vi "Check Condition.vi"(1 "Distance":dbl, 2 "Condition":dbl, 3 "Reset":bool) -> (0 "Done":bool)   [LabVIEW 2015]
uses:
  Robot Global Data.vi
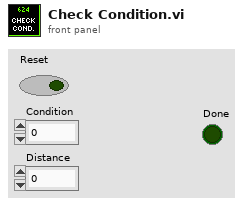
[diagram p1: front panel]
types:
  T1 = typedef "Encoder Values Super Cluster.ctl" = cluster{"Left Encoder":T2, "Right Encoder":T2}
  T2 = typedef "Encoder Values.ctl" = cluster{"Distance":dbl, "Speed":dbl, "Ticks":dbl}
  T3 = typedef "Dashboard Control Data.ctl" = cluster{"Shooter Presets":T4, "Encoder Control":T6, "Steer PID output":cluster{"output high":dbl, "output low":dbl}, " Steer PID gains":cluster{"proportional gain (Kc)":dbl, "integral time (Ti, min)":dbl, "derivative time (Td, min)":dbl}, "Drivetrain Settings":T7, "Vision Packet":T8, "Dashboard Drivetrain Command":T9, "Info/Command Cluster":T11, "Ball Vision Packet":T12, "Intake Presets":T14, "Intake Encoder Control":T16, "Climb Presets":T17, "Goal Output Range":cluster{"output high":dbl, "output low":dbl}, "Enabled Systems":T18, "Auton Presets":T19, "Pressure M":dbl, "Pressure B":dbl, "Vision Timeout":dbl}
  T4 = typedef "Shooter Presets.ctl" = cluster{"Batter Shot":T5, "Deep Middle":T5, "Manual Shot":T5, "Left Ticks Per Rotation":dbl, "Right Ticks Per Rotation":dbl, "Low Bar Shot":T5, "Shooter RPM Tolerance":dbl, "Trigger Power":dbl, "Fire from Load Delay":i32, "Max Angle":dbl, "Min Angle":dbl, "Angle PID gains":cluster{"P":dbl, "I":dbl, "D":dbl}, "Angle Output":cluster{"output high":dbl, "output low":dbl}, "Shooter Angle Tolerance":dbl, "Vision Shoot x^2":dbl, "Vision Shoot x":dbl, "Feed Forward Max Accel":dbl, "Feed Forward Kv":dbl, "Backwards Trigger":dbl, "Shot Finish Delay (ms)":dbl, "Angle Max Current":dbl, "Angle Current Trip Time":dbl, "Intake Angle":dbl, "Vision Shoot c":dbl, "Reset?":bool, "Button Release Delay":dbl, "Angle Pot x":dbl, "Angle Pot c":dbl, "Ignore Angle?":bool, "Max RPM":dbl, "Safty Frist Angle":dbl, "Intake Danger Height":dbl, "Angle Pot B":i32, "Angle Pot M":dbl, "FF Finish RPM":dbl, "RPM PID Right":cluster{"P":dbl, "I":dbl, "D":dbl, "FF":dbl}, "RPM PID Left":cluster{"P":dbl, "I":dbl, "D":dbl, "FF":dbl}, "Backwards RPM":dbl, "Vision RPM":dbl, "Run Wheels Backward Delay":u32, "Cleat Shot":T5}
  T5 = typedef "Shot Presets.ctl" = cluster{"L":dbl, "R":dbl, "A":dbl}
  T6 = typedef "Encoder Control.ctl" = cluster{"Right Tick Constant":dbl, "Left Tick Constant":dbl, "Reset?":bool, "Y Dist":cluster{"PID gains":cluster{"proportional gain (Kc)":dbl, "integral time (Ti, min)":dbl, "derivative time (Td, min)":dbl}}, "Y Stop Thresh":dbl, "Y Stop Speed":dbl}
  T7 = typedef "Drivetrain Settings.ctl" = cluster{"Gyro Tolerance":dbl, "Throttle Ramp (ms)":dbl, "Kv":dbl, "Ka":dbl, "Feed Forward P":dbl, "Feed Forward D":dbl, "Goal Vision PID gains":cluster{"proportional gain (Kc)":dbl, "integral time (Ti, min)":dbl, "derivative time (Td, min)":dbl}, "Goal Detection Window":dbl, "Creep Rate":dbl, "Vision Throttle Threshold":dbl, "Min Turn Output":dbl, "Left Batter Angle":dbl, "Right Batter Angle":dbl}
  T8 = typedef "Goal Vision Packet.ctl" = cluster{"Distance":dbl, "Center X":dbl, "Center Y":dbl, "Found Target?":bool, "Robot Center":dbl, "Angle":dbl}
  T9 = typedef "Dashboard Drivetrain Command.ctl" = cluster{"Drivetrain Vision":T10}
  T10 = typedef "Drivetrain Vision.ctl" = cluster{"Goal Window":dbl, "Ball Window":dbl}
  T11 = typedef "Ball Tracking Command Cluster.ctl" = cluster{"Distance to Ball":dbl, "Desired Angle":dbl, "Command":enum16{"Turn to Ball", "Turn to Angle", "Get Distance"}, "Pixels from Center":dbl}
  T12 = typedef "Ball Vision Packet.ctl" = cluster{"Ball Detected?":bool, "Distance to Ball":dbl, "Desired Angle":dbl, "Pixels from Center":dbl, "Tracking mode":T13}
  T13 = typedef "Tracking Mode.ctl" = enum16{"Turn to Ball", "Turn to Angle"}
  T14 = typedef "Intake Presets.ctl" = cluster{"Intake Speed":dbl, "Outake Speed":dbl, "Low Height":dbl, "Half Height":dbl, "Full Height":dbl, "Angle Speed":dbl, "Angle Tolerance":dbl, "Encoder Scale":dbl, "Load Height":dbl, "Output Range":T15, "Rotation Power Max/Min":dbl, "MaxCurrent":dbl, "Intake Trip Time":dbl, "Idle Height":dbl, "Max Height":dbl, "Reset Encoders?":bool, "PID gains":cluster{"proportional gain (Kc)":dbl, "integral time (Ti, min)":dbl, "derivative time (Td, min)":dbl}, "Intake Stop Delay":u32, "Settle Time":dbl, "Settle Wait Time":dbl}
  T15 = typedef "Drivetrain Output Range.ctl" = cluster{"output high":dbl, "output low":dbl}
  T16 = typedef "IntakeEcoderControl.ctl" = cluster{"Arm Tick Constant":dbl, "Reset?":bool, "Y Dist":cluster{"PID gains":cluster{"proportional gain (Kc)":dbl, "integral time (Ti, min)":dbl, "derivative time (Td, min)":dbl}}, "Y Stop Thresh":dbl, "Y Stop Speed":dbl}
  T17 = typedef "Climb Presets.ctl" = cluster{"Pull Power":dbl, "Extend Power":dbl}
  T18 = typedef "Enabled Systems.ctl" = cluster{"Shoot":bool, "Intake":bool, "DT":bool, "Gyro":bool, "100ms":bool, "US":bool}
  T19 = typedef "Autonomous Presets.ctl" = cluster{"Pitch Limit":dbl, "Roll Limit":dbl, "Start Position":dbl, "Cross Position":dbl}
  T20 = typedef "IMU Data.ctl" = cluster{"Pitch":sgl, "Roll":sgl, "Yaw":sgl, "Data Valid?":bool, "Temp":sgl, "MOVING":bool, "YAW_STABLE":bool, "Accel X":sgl, "Accel Y":sgl, "Accel Z":sgl, "Accel Magnitude":sgl, "Pitch Rate":sgl, "Roll Rate":sgl, "Yaw Rate":sgl, "NavX Opened?":bool, "Calibration Status":T21, "OP Status":T22}
  T21 = typedef "navX Library v2.lvlib/Z900_navX_Flags_CalibrationStatusTypeDef.ctl" = u8
  T22 = typedef "navX Library v2.lvlib/Z900_navX_Flags_OpStatusTypeDef.ctl" = u8
  T23 = typedef "Drivetrain Status Cluster.ctl" = cluster{"Modes":T24, "Y (Throttle)":dbl, "X (Steer)":dbl, "Gyro In Range?":bool, "Distance Drive Finished?":bool, "Stop Eject Lockout":bool, "Dist Drive Status":T25, "Y Target":dbl, "Heading Target":dbl, "Vision Target Aligned?":bool, "Gear":dbl, "1st Gear Time":dbl, "2nd Gear Time":dbl, "1st Gear Shifts":dbl, "2nd Gear Shifts":dbl}
  T24 = typedef "Drivetrain Modes.ctl" = enum16{"Tank", "Climb", "Manual", "Goal Vision Targeting", "PID Distance Drive", "Hybrid", "Gyro Steer"}
  T25 = typedef "Dist Drive Status.ctl" = cluster{"Y In Range":bool, "X In Range":bool, "Gyro In Range":bool, "Y Dist":dbl, "X Dist":dbl, "Gyro":dbl}
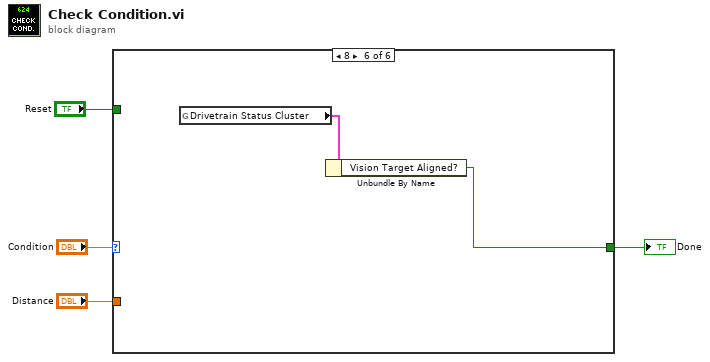
[diagram p0: block diagram]
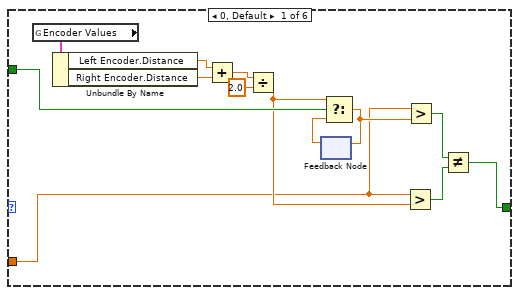
[diagram p2: hidden frame]
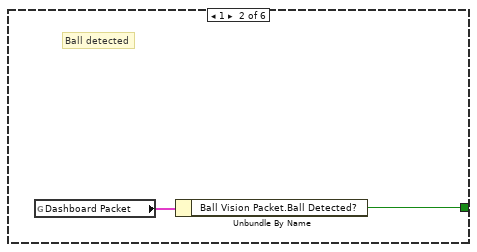
[diagram p3: hidden frame]
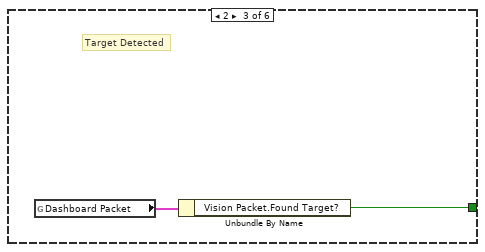
[diagram p4: hidden frame]
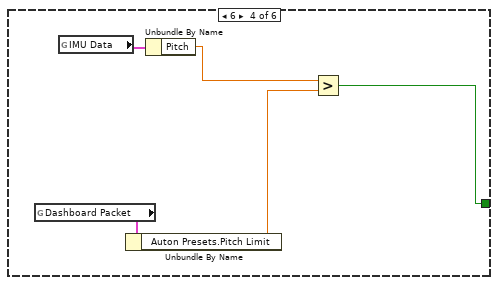
[diagram p5: hidden frame]
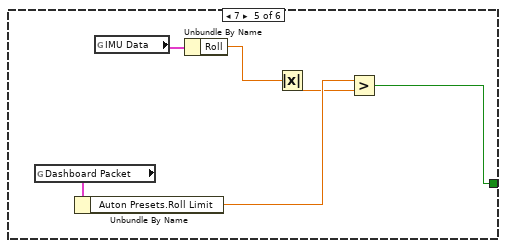
[diagram p6: hidden frame]
diagram:
  n1 = case shown="8" "Condition" {
    tunnel: "Distance" -> [w8 _ _ _ _ _]
    tunnel: "Reset" -> [w12 _ _ _ _ _]
    tunnel: [w5 w18 w20 w22 w29 w33] -> w1
    frame 0, Default {
      n2 = global read "Robot Global Data.vi" "Encoder Values"() -> (w17:T1)
      n3 = Unbundle By Name(w17) -> ("Left Encoder.Distance"=w16:dbl, "Right Encoder.Distance"=w15:dbl)
      n4 = Add(x=w16, y=w15) -> (x+y=w14:dbl)
      n5 = Divide(x=w14, y=2.0) -> (x/y=w9:dbl)
      n6 = feedback #1() -> (w11:dbl)  [unwired: 1 in]
      n7 = Select(t=w9, s=w12, f=w11) -> (s? t:f=w10:dbl)
      n8 = feedback-in #1(w10) -> ()
      n9 = Greater?(x=w8, y=w9) -> (0:w6:bool)
      n10 = Greater?(x=w8, y=w10) -> (0:w7:bool)
      n11 = Not Equal?(x=w7, y=w6) -> (x != y?=w5:bool)
    }
    frame 1 {
      # "Ball detected"
      n12 = global read "Robot Global Data.vi" "Dashboard Packet"() -> (w19:T3)
      n13 = Unbundle By Name(w19) -> ("Ball Vision Packet.Ball Detected?"=w18:bool)
    }
    frame 2 {
      # "Target Detected"
      n14 = global read "Robot Global Data.vi" "Dashboard Packet"() -> (w21:T3)
      n15 = Unbundle By Name(w21) -> ("Vision Packet.Found Target?"=w20:bool)
    }
    frame 6 {
      n16 = global read "Robot Global Data.vi" "Dashboard Packet"() -> (w26:T3)
      n17 = global read "Robot Global Data.vi" "IMU Data"() -> (w25:T20)
      n18 = Unbundle By Name(w26) -> ("Auton Presets.Pitch Limit"=w23:dbl)
      n19 = Unbundle By Name(w25) -> ("Pitch"=w24:sgl)
      n20 = Greater?(x=w24, y=w23) -> (0:w22:bool)
    }
    frame 7 {
      n21 = global read "Robot Global Data.vi" "Dashboard Packet"() -> (w32:T3)
      n22 = Unbundle By Name(w32) -> ("Auton Presets.Roll Limit"=w30:dbl)
      n23 = global read "Robot Global Data.vi" "IMU Data"() -> (w31:T20)
      n24 = Unbundle By Name(w31) -> ("Roll"=w28:sgl)
      n25 = Absolute Value(x=w28) -> (abs(x)=w27:sgl)
      n26 = Greater?(x=w30, y=w27) -> (0:w29:bool)
    }
    frame 8 {
      n27 = global read "Robot Global Data.vi" "Drivetrain Status Cluster"() -> (w34:T23)
      n28 = Unbundle By Name(w34) -> ("Vision Target Aligned?"=w33:bool)
    }
  }
  "Done" <- w1
